vi "LEDRincController.vi"() -> ()   [LabVIEW 2024]
uses:
  <vilib>/Instr/_visa.llb/VISA Configure Serial Port (Instr).vi
panel:
  in  "stop 5":bool
  in  "Enum":enum16{"Idle", "Off", "Block", "Access"}(ring)
  in  "Port":refnum<visa-resource-name>
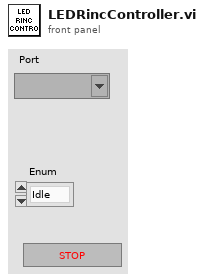
[diagram p1: front panel]
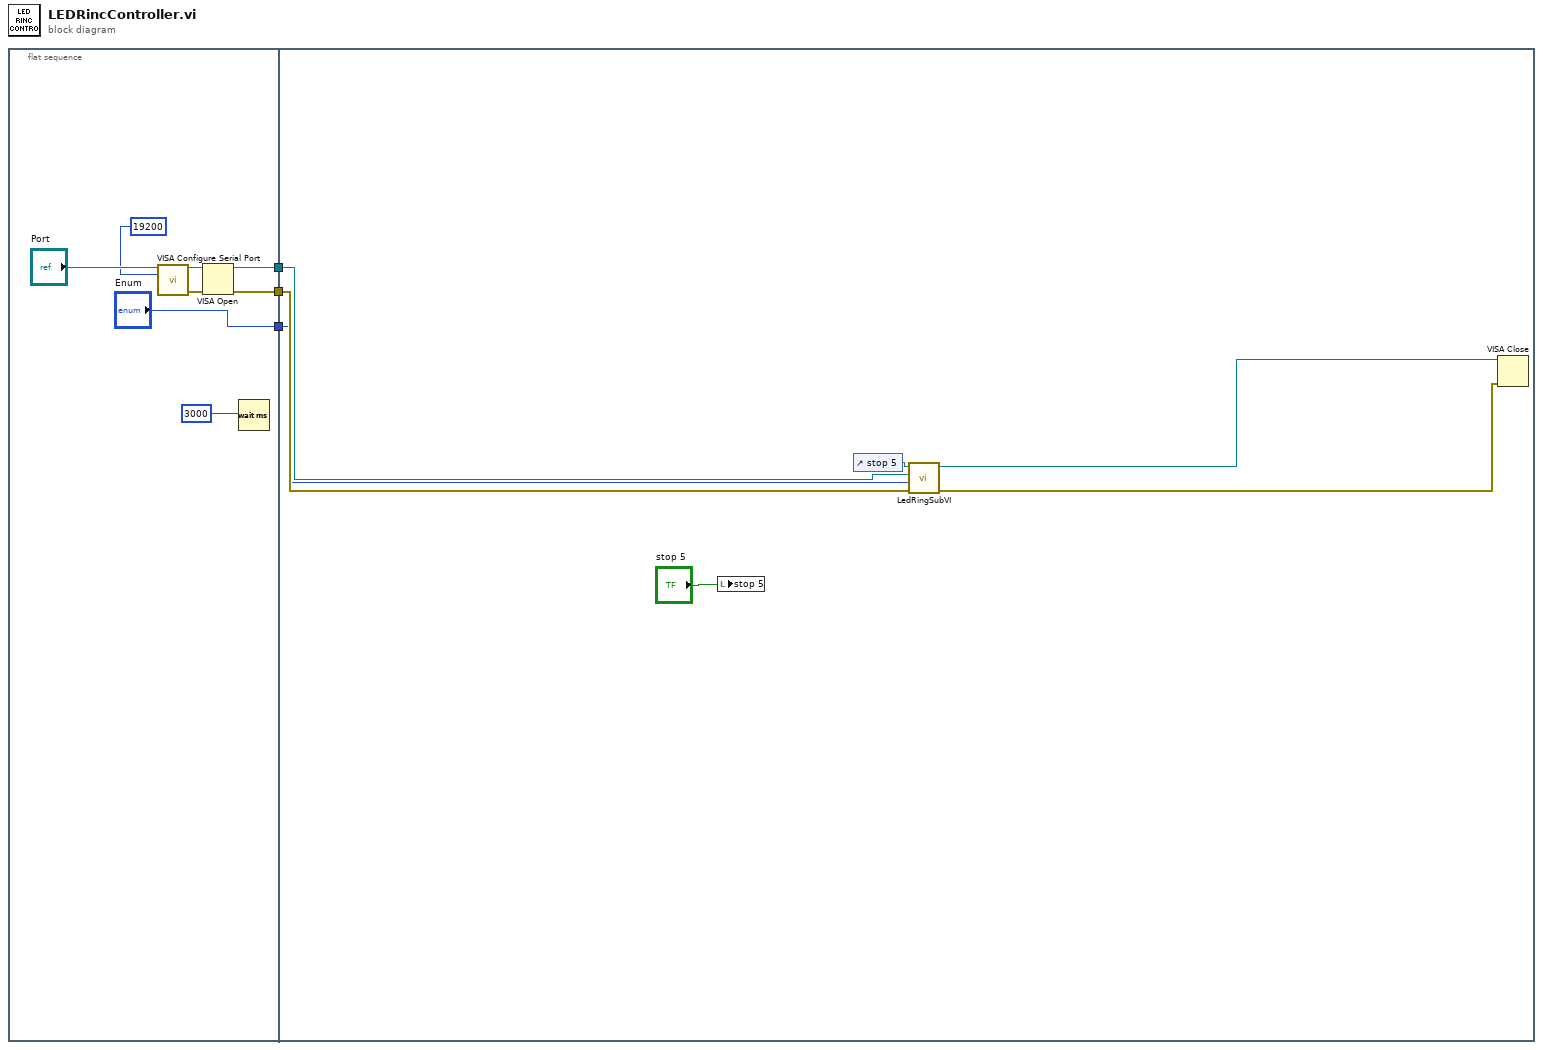
[diagram p0: block diagram]
diagram:
  n1 = flat-sequence {
    tunnel: ["Enum"] -> w3
    tunnel: [w6] -> w2
    tunnel: [w5] -> w1
    tunnel: w3 -> [w14]
    tunnel: w2 -> [w18]
    tunnel: w1 -> [w17]
    frame #0 {
      n2 = call-poly "VISA Configure Serial Port"("VISA resource name"="Port", "baud rate (9600)"=u32 19200) -> ("VISA resource name out"=w10:refnum<visa-resource-name>, "error out"=w9:errorcluster)  [unwired: 12 in]
      n3 = VISA Open(error in (no error)=w9, VISA resource name=w10) -> (VISA resource name=w6:refnum<visa-resource-name>, error out=w5:errorcluster)  [unwired: 3 in]
      n4 = Wait (ms)(milliseconds to wait=u32 3000 ("millisecond multiple")) -> ()  [unwired: 1 out]
    }
    frame #1 {
      n5 = local write "stop 5"("stop 5") -> ()
      n6 = control-ref of="stop 5"() -> (w12:refnum<vi>)
      n7 = call "LedRingSubVI.vi"("error in (no error)"=w17, "Enum"=w14, "VISA resource name in"=w18, "Boolean in"=w12) -> ("error out"=w16:errorcluster, "VISA Refnum out"=w15:refnum<visa-resource-name>)  [unwired: 6 in]
      n8 = VISA Close(VISA resource name=w15, error in (no error)=w16) -> ()  [unwired: 1 out]
    }
  }
